vi "Synchio.Initialize.vi"(8 "error in (no error)":errorcluster, 10 "AI/AO Config":T1={"AI Configuration"=[], "AO Configuration"=[], "sampling info"={"Fs"=0.0, "#s"=0.0}, "AO"={"AO amp (V)"=[0.1, 0.09, 0.08, 0.07, 0.06, 0.05, 0.04, 0.03], "AO DC (V)"=[0.0, 0.0, 0.0, 0.0, 0.0, 0.0, 0.0, 0.0], "AO f (Hz)"=[13.0, 13.0, 13.0, 13.0, 13.0, 13.0, 13.0, 13.0], "AO phi (deg)"=[0.0, 0.0, 0.0, 0.0, 0.0, 0.0, 0.0, 0.0], "function"=[enum."Sine Wave", enum."Sine Wave", enum."Sine Wave", enum."Sine Wave", enum."Sine Wave", enum."Sine Wave", enum."Sine Wave", enum."Sine Wave"]}} {"AO"."AO DC (V)" format="%#_6p"; "AO"."AO amp (V)" format="%#_6p"}, 11 "SynchIO.USB4431 in":refnum<class "SynchIO.USB4431.lvclass">) -> (0 "error out":errorcluster, 1 "AO Task":refnum<k21>[](array[refnum]), 2 "AI task":refnum<k21>[](array[refnum]), 3 "SynchIO.USB4431 out":refnum<class "SynchIO.USB4431.lvclass">)   [LabVIEW 2016, in "SynchIO.USB4431.lvclass"]
uses:
  SynchIO.USB4431.lvclass
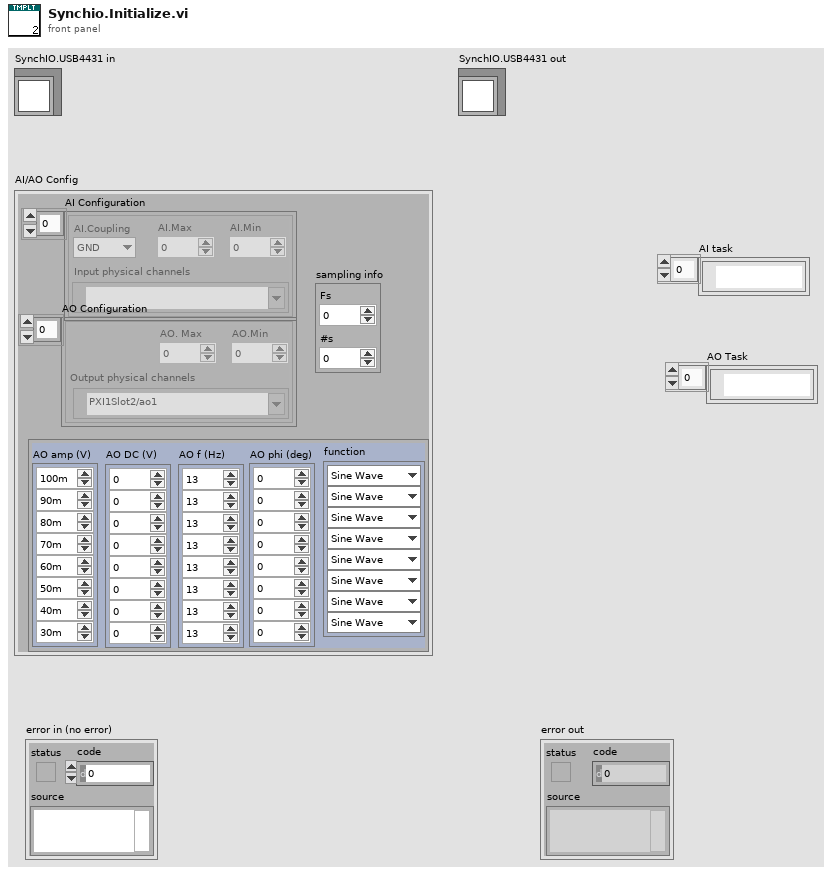
[diagram p1: front panel]
types:
  T1 = cluster{"AI Configuration":cluster{"AI.Coupling":enum16{"AC", "DC", "GND"}, "AI.Max":dbl, "AI.Min":dbl, "Input physical channels":tag}[], "AO Configuration":cluster{"Output physical channels":tag, "AO. Max":dbl, "AO.Min":dbl}[], "sampling info":cluster{"Fs":dbl, "#s":dbl}, "AO":cluster{"AO amp (V)":dbl[], "AO DC (V)":dbl[], "AO f (Hz)":dbl[], "AO phi (deg)":dbl[], "function":enum16{"Sine Wave", "Triangle Wave", "Square Wave", "Sawtooth Wave"}[]}}
  T2 = cluster{"AI.Coupling":enum16{"AC", "DC", "GND"}, "AI.Max":dbl, "AI.Min":dbl, "Input physical channels":tag}[]
  T3 = cluster{"Output physical channels":tag, "AO. Max":dbl, "AO.Min":dbl}[]
  T4 = cluster{"AO amp (V)":dbl[], "AO DC (V)":dbl[], "AO f (Hz)":dbl[], "AO phi (deg)":dbl[], "function":enum16{"Sine Wave", "Triangle Wave", "Square Wave", "Sawtooth Wave"}[]}
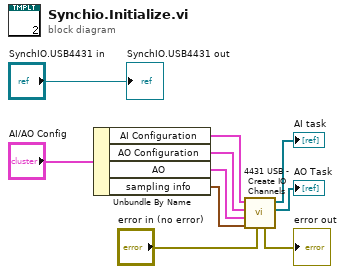
[diagram p0: block diagram]
diagram:
  n1 = Unbundle By Name("AI/AO Config") -> ("AI Configuration"=w9:T2, "AO Configuration"=w8:T3, "AO"=w7:T4, "sampling info"=w6:cluster{"Fs":dbl, "#s":dbl})
  n2 = call "4431 USB - Create IO Channels.vi"("error in"="error in (no error)", "sampling info"=w6, "AO"=w7, "AO Configuration"=w8, "AI Configuration"=w9) -> ("AO Task"=→"AO Task":refnum<k21>[], "AI task"=→"AI task":refnum<k21>[], "error out"=→"error out":errorcluster)  [unwired: 4 in]
  "SynchIO.USB4431 out" <- "SynchIO.USB4431 in"
